vi "ws_authenticate user credentials.vi"(4 "Session Timeout, Seconds (0)":i32, 5 "Attempts (0)":i32, 6 "Force Logout? (f)":bool, 7 "REMOTE_ADDR (\"\")":string, 8 "error in (no error)":errorcluster, 9 "Passhash (\"\")":string, 10 "Username (\"\")":string, 11 "DB Connection Ref":T2) -> (0 "error out":errorcluster, 2 "User Record":T1, 3 "User must login?":bool)   [LabVIEW 2011]
uses:
  SI.LIB/ODBC/SQL Controls/Connection Refnum.ctl
  server/database/Users/User Record.ctl
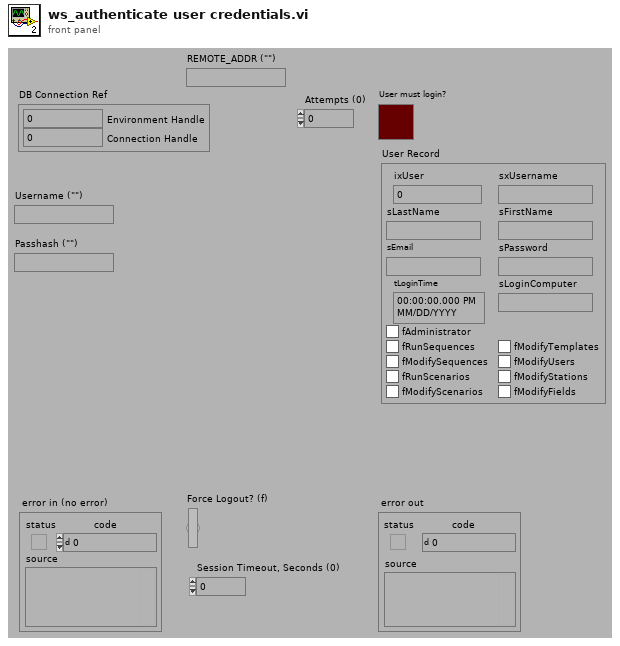
[diagram p1: front panel]
types:
  T1 = typedef "User Record.ctl" = cluster{"ixUser":i32, "sxUsername":string, "sLastName":string, "sFirstName":string, "sEmail":string, "sPassword":string, "tLoginTime":timestamp, "sLoginComputer":string, "fAdministrator":bool, "fRunSequences":bool, "fModifySequences":bool, "fRunScenarios":bool, "fModifyScenarios":bool, "fModifyTemplates":bool, "fModifyUsers":bool, "fModifyStations":bool, "fModifyFields":bool}
  T2 = typedef "Connection Refnum.ctl" = cluster{"Environment Handle":i32, "Connection Handle":i32}
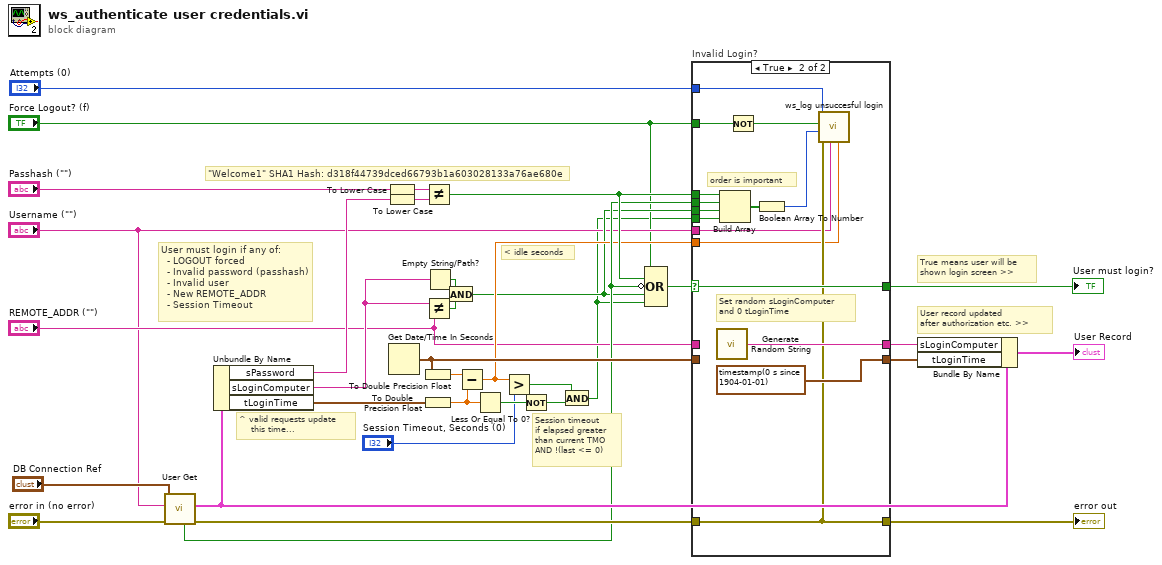
[diagram p0: block diagram]
diagram:
  # "< idle seconds"
  # "Session timeout\nif elapsed greater\nthan current TMO\nAND !(last <= 0)"
  # "^ valid requests update\n    this time..."
  # "User must login if any of:\n  - LOGOUT forced\n  - Invalid password (passhash)\n  - Invalid user\n  - New REMOTE_ADDR\n  - Session Timeout"
  # "\"Welcome1\" SHA1 Hash: d318f44739dced66793b1a603028133a76ae680e"
  # "User record updated\nafter authorization etc. >>"
  # "True means user will be \nshown login screen >>"
  n1 = call "User Get.vi"("error in (no error)"="error in (no error)", "sxUsername (\"\")"="Username (\"\")", "Connection Refnum"="DB Connection Ref") -> ("error out"=w28:errorcluster, "User"=w34:T1, "Data Present?"=w26:bool)  [unwired: 6 out]
  n2 = Unbundle By Name(w34) -> ("sPassword"=w29:string, "sLoginComputer"=w22:string, "tLoginTime"=w21:timestamp)
  n3 = To Lower Case(string="Passhash (\"\")") -> (all lower case string=w24:string)
  n4 = To Lower Case(string=w29) -> (all lower case string=w23:string)
  n5 = Get Date/Time In Seconds() -> (seconds since 1Jan1904=w30:timestamp)
  n6 = To Double Precision Float(number=w30) -> (double precision float=w20:dbl)
  n7 = To Double Precision Float(number=w21) -> (double precision float=w6:dbl)
  n8 = Not Equal?(x=w24, y=w23) -> (x != y?=w27:bool)
  n9 = Not Equal?(x=w22, y="REMOTE_ADDR (\"\")") -> (x != y?=w18:bool)
  n10 = Empty String/Path?(string/path=w22) -> (empty?=w19:bool)
  n11 = And(x=w19, y=w18) -> (x .and. y?=w17:bool)
  n12 = Subtract(x=w20, y=w6) -> (x-y=w25:dbl)
  n13 = Less Or Equal To 0?(x=w6) -> (x <= 0?=w5:bool)
  n14 = Greater?(x=w25, y="Session Timeout, Seconds (0)") -> (0:w4:bool)
  n15 = Not(x=w5) -> (.not. x?=w1:bool)
  n16 = And(x=w4, y=w1) -> (x .and. y?=w3:bool)
  n17 = Compound Arithmetic op=OR("Force Logout? (f)", w27, invert w26, w17, w3) -> (w31:bool)
  n18 = case "Invalid Login?" shown="True" w31 {
    selector: w31 -> [w38 w53]
    tunnel: [w38 w53] -> w12
    tunnel: [w37 timestamp(0 s since 1904-01-01) ("tLoginTime")] -> w33
    tunnel: [w36 w51] -> w32
    tunnel: w30 -> [w37 _]
    tunnel: "REMOTE_ADDR (\"\")" -> [w36 _]
    tunnel: w28 -> [w35 w50]
    tunnel: [w35 w50] -> w15
    tunnel: "Force Logout? (f)" -> [_ w42]
    tunnel: w27 -> [_ w47]
    tunnel: w26 -> [_ w46]
    tunnel: w17 -> [_ w45]
    tunnel: w3 -> [_ w44]
    tunnel: w25 -> [_ w48]
    tunnel: "Username (\"\")" -> [_ w40]
    tunnel: "Attempts (0)" -> [_ w39]
    frame False {
    }
    frame True {
      # "order is important"
      # "Set random sLoginComputer\nand 0 tLoginTime"
      n19 = call "Generate Random String.vi"() -> ("Output String"=w51:string)  [unwired: 1 in, 4 out]
      n20 = Build Array(w47, w46, w45, w44) -> (w43:bool[])
      n21 = Not(x=w42) -> (.not. x?=w41:bool)
      n22 = Boolean Array To Number(Boolean array=w43) -> (number=w49:u32)
      n23 = call "ws_log unsuccesful login.vi"("session time (0.00)"=w48, "username (\"\")"=w40, "error in (no error)"=w50, "Bad Bits (0)"=w49, "Log Bad Attempt? (f)"=w41, "Attempts (\"\")"=w39) -> ()  [unwired: 5 in, 1 out]
    }
  }
  "error out" <- w15
  "User must login?" <- w12
  n24 = Bundle By Name(cluster=w34, "sLoginComputer"=w32, "tLoginTime"=w33) -> (→"User Record":T1)
